vi "AlliGator Parameter Names to Parameters List.vi"(11 "Parameter Names":string[](array[string])) -> (1 "Complete Map":bool, 3 "[Decay Fit Parameter Name]":T1[](array[typedef]))   [LabVIEW 2021, in "AlliGator Python Plugins.lvlib"]
doc: "Converts parameter names to an array of enums."
uses:
  AlliGator Python Plugins.lvlib
  Fits/IRF(X)PSED/Decay Fit Parameters & Derived Quantities List.ctl
  Fits/Fits.lvlib
panel:
  # "see the AlliGator License on the block diagram (Ctrl+E or Window:Show Block Diagram)"
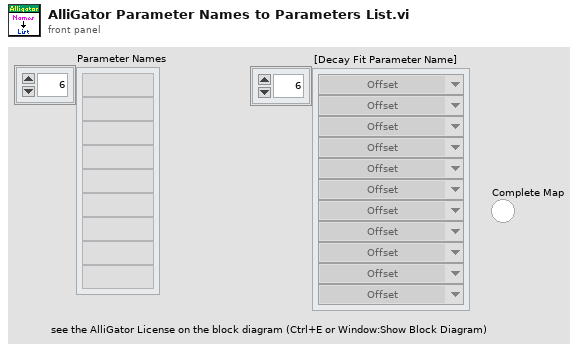
[diagram p1: front panel]
types:
  T1 = typedef "Fits.lvlib/Decay Fit Parameters & Derived Quantities List.ctl" = enum16{"Offset", "Baseline", "A_1", "tau_1", "A_2", "tau_2", "<tau>_a", "f1_a", "f2_a", "<tau>_i", "f1_i", "f2_i", "-", "R^2", "Chi^2"}
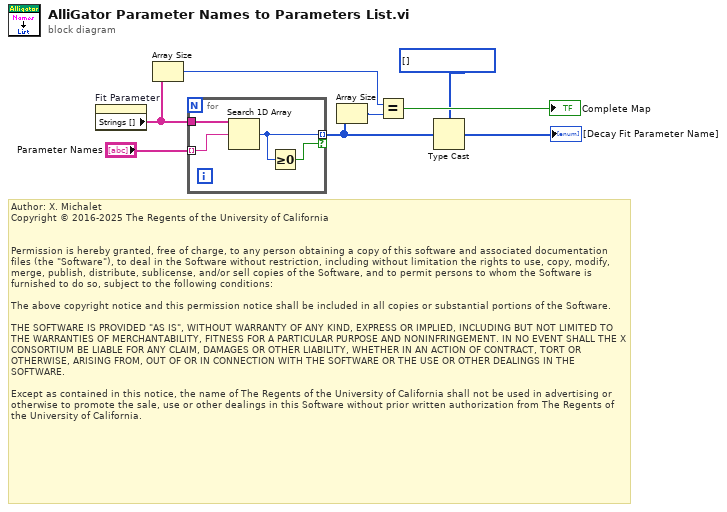
[diagram p0: block diagram]
diagram:
  w1 = T1[] [] items=["Offset", "Baseline", "A_1", "tau_1", "A_2", "tau_2", "<tau>_a", "f1_a", "f2_a", "<tau>_i", "f1_i", "f2_i", "-", "R^2", "Chi^2"] ("[Decay Fit Parameter Name]")
  # "Author: X. Michalet\nCopyright © 2016-2025 The Regents of the University of California\n \n\nPermission is hereby granted, free of charge, to any person obtaining a copy of this software and associated documentation files (the \"Software\"), to deal in the Software without restriction, including without limitation the rights to use, copy, modify, merge, publish, distribute, sublicense, and/or sell copies of the Software, and to permit persons to whom the Software is furnished to do so, subject to the following conditions:\n\nThe above copyright notice and this permission notice shall be included in all copies or substantial portions of the Software.\n\nTHE SOFTWARE IS PROVIDED \"AS IS\", WITHOUT WARRANTY OF ANY KIND, EXPRESS OR IMPLIED, INCLUDING BUT NOT LIMITED TO THE WARRANTIES OF MERCHANTABILITY, FITNESS FOR A PARTICULAR PURPOSE AND NONINFRINGEMENT. IN NO EVENT SHALL THE X CONSORTIUM BE LIABLE FOR ANY CLAIM, DAMAGES OR OTHER LIABILITY, WHETHER IN AN ACTION OF CONTRACT, TORT OR OTHERWISE, ARISING FROM, OUT OF OR IN CONNECTION WITH THE SOFTWARE OR THE USE OR OTHER DEALINGS IN THE SOFTWARE.\n\nExcept as contained in this notice, the name of The Regents of the University of California shall not be used in advertising or otherwise to promote the sale, use or other dealings in this Software without prior written authorization from The Regents of the University of California."
  n1 = property on="Fit Parameter" class="Enum (strict)"() -> ("Strings []"=w7:string[])  [unwired: 2 in, 2 out]
  n2 = Array Size(array=w7) -> (size(s)=w4:i32)
  n3 = for {
    tunnel: "Parameter Names" -> [w11] mode=indexing
    tunnel: w7 -> [w12]
    tunnel: [w10] -> w6 mode=indexing if=w9
    n4 = Search 1D Array(1D array=w12, element=w11) -> (index of element=w10:i32)  [unwired: 1 in]
    n5 = Greater Or Equal To 0?(x=w10) -> (x >= 0?=w9:bool)
  }
  n6 = Array Size(array=w6) -> (size(s)=w5:i32)
  n7 = Equal?(x=w4, y=w5) -> (x = y?=→"Complete Map":bool)
  n8 = Type Cast(type=w1, x=w6) -> (*(type *) &x=→"[Decay Fit Parameter Name]":T1[])
